vi "20T_Go_To_Set.vi"(8 "error in (no error)":errorcluster, 10 "20T Control":T1={"Clamp"=TRUE, "Switch Heater"=TRUE, "Go to Zero"=TRUE, "Go to Set"=FALSE, "Go to Hold"=FALSE, "Field Setpoint (T)"=3.4572, "Rate Setpoint (T/min)"=0.0, "Set Rate"=FALSE, "Activate lambda control"=FALSE, "Set lambda NV"=FALSE, "lambda NV  SP"=3.4572} {"lambda NV  SP" format="%.1f"; "Rate Setpoint (T/min)" format="%6_5f"; "Field Setpoint (T)" format="%#4_5f"}, 11 "Mercury Reference In":T2) -> (0 "error out":errorcluster)   [LabVIEW 2019]
uses:
  Equipment/Mercury iXX/Public/Controls/Mercury Reference.ctl
  Equipment/Mercury iXX/Public/Controls/Comms Transport Layer.ctl
  Equipment/Mercury iXX/Private/Controls/Query Dynamic Reference.ctl
  Monitor Communication/Gustav/20T_Control.ctl
  Global/Global Variables/Data_Display_global.vi
  Equipment/Mercury iXX/Public/Libraries/Magnet/Open/Open Magnet Device.vi
  Monitor Communication/sub-vis/20T_Open_Queue.vi
  Monitor Communication/sub-vis/20T_Queue_Commands.vi
  Equipment/Mercury iXX/Mercury iXX.lvlib
  Equipment/Mercury iXX/Public/Libraries/Magnet.lvlib
panel:
  # "20 T"
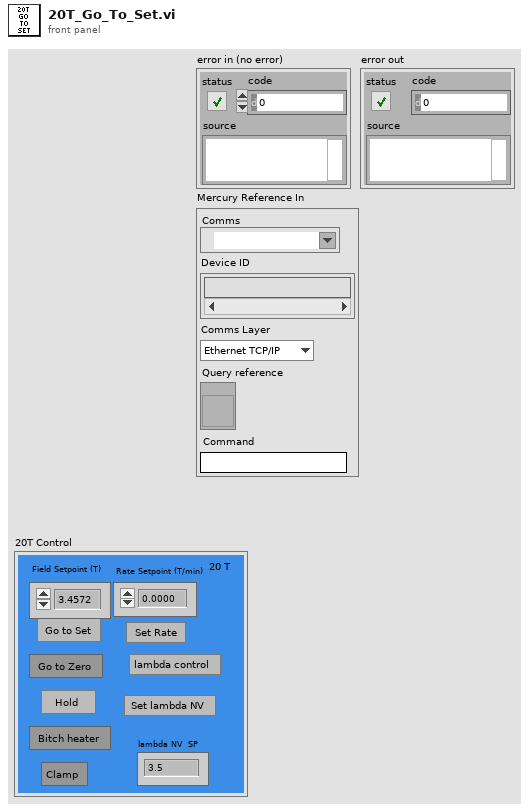
[diagram p1: front panel]
types:
  T1 = typedef "20T_Control.ctl" = cluster{"Clamp":bool, "Switch Heater":bool, "Go to Zero":bool, "Go to Set":bool, "Go to Hold":bool, "Field Setpoint (T)":dbl, "Rate Setpoint (T/min)":dbl, "Set Rate":bool, "Activate lambda control":bool, "Set lambda NV":bool, "lambda NV  SP":dbl}
  T2 = typedef "Mercury iXX.lvlib/Mercury Reference.ctl" = cluster{"Comms":refnum<visa-resource-name>, "Device ID":string[], "Comms Layer":T3, "Command":string, "Query reference":T4}
  T3 = typedef "Mercury iXX.lvlib/Comms Transport Layer.ctl" = enum16{"Ethernet TCP/IP", "USB", "ISOBus - RS-232", "GPIB"}
  T4 = typedef "Mercury iXX.lvlib/Query Dynamic Reference.ctl" = refnum<vi>
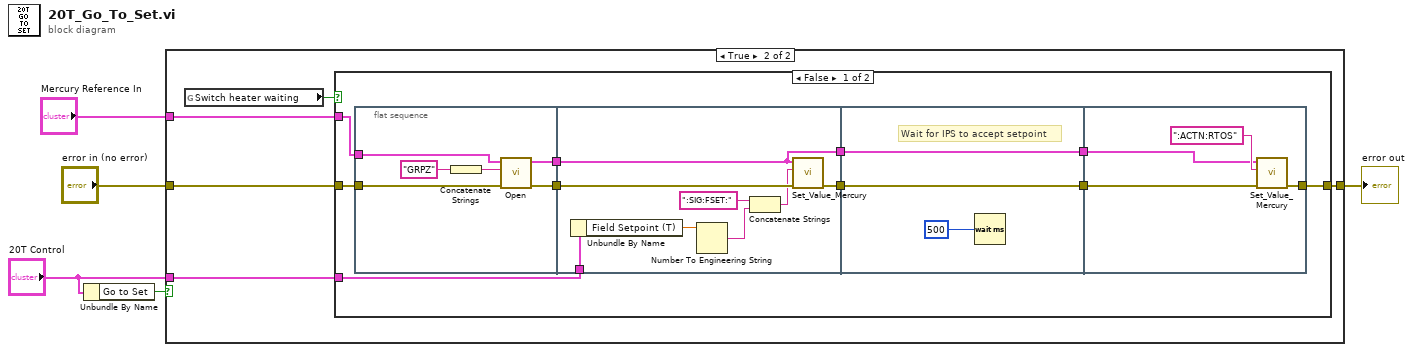
[diagram p0: block diagram]
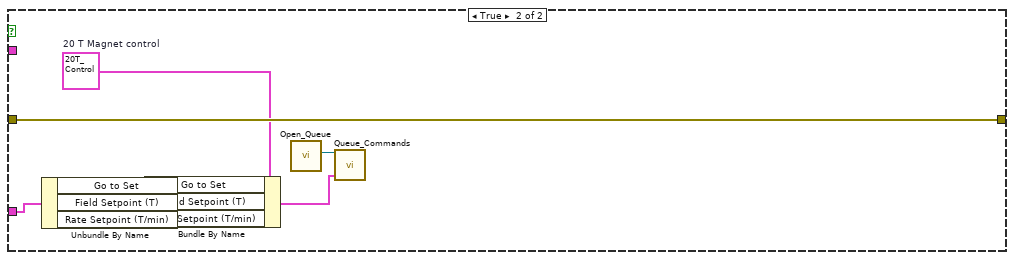
[diagram p3: hidden frame]
diagram:
  n1 = Unbundle By Name("20T Control") -> ("Go to Set"=w4:bool)
  n2 = case shown="True" w4 {
    tunnel: [w6 w7] -> w5
    tunnel: "20T Control" -> [_ w10]
    tunnel: "Mercury Reference In" -> [_ w9]
    tunnel: "error in (no error)" -> [w6 w8]
    frame False {
    }
    frame True {
      n3 = global read "Data_Display_global.vi" "Switch heater waiting"() -> (w11:bool)
      n4 = case shown="False" w11 {
        tunnel: [w21 w49] -> w7
        tunnel: w10 -> [w20 w48]
        tunnel: w9 -> [w17 _]
        tunnel: w8 -> [w16 w49]
        frame False {
          n5 = flat-sequence {
            tunnel: [w22] -> w19
            tunnel: [w23] -> w18
            tunnel: w17 -> [w25]
            tunnel: w16 -> [w24]
            tunnel: [w31] -> w15
            tunnel: [w33] -> w13
            tunnel: w20 -> [w28]
            tunnel: w19 -> [w32]
            tunnel: w18 -> [w33]
            tunnel: w15 -> [w38]
            tunnel: [w38] -> w14
            tunnel: w13 -> [w37]
            tunnel: [w37] -> w12
            tunnel: [w41] -> w21
            tunnel: w14 -> [w39]
            tunnel: w12 -> [w40]
            frame #0 {
              n6 = Concatenate Strings("GRPZ" ("Device Identifier")) -> (w27:string)
              n7 = call-poly "Open.vi"("error in (no error)"=w24, "Device Identifier"=w27, "Mercury Reference In"=w25) -> ("error out"=w22:errorcluster, "Mercury Reference Out"=w23:T2)  [unwired: 1 in, 6 out]
            }
            frame #1 {
              n8 = Unbundle By Name(w28) -> ("Field Setpoint (T)"=w29:dbl)
              n9 = Number To Engineering String(4:w29) -> (0:w35:string)  [unwired: 3 in]
              n10 = Concatenate Strings(":SIG:FSET:", w35) -> (w30:string)
              n11 = call "Set_Value_Mercury.vi"("error in"=w32, "Noun(s)"=w30, "Mercury Reference In"=w33) -> ("error out"=w31:errorcluster)  [unwired: 7 in, 1 out]
            }
            frame #2 {
              # "Wait for IPS to accept setpoint"
              n12 = Wait (ms)(milliseconds to wait=500) -> ()  [unwired: 1 out]
            }
            frame #3 {
              n13 = call "Set_Value_Mercury.vi"("error in"=w39, "Noun(s)"=":ACTN:RTOS", "Mercury Reference In"=w40) -> ("error out"=w41:errorcluster)  [unwired: 7 in, 1 out]
            }
          }
        }
        frame True {
          w47 = T1 {"Clamp"=FALSE, "Switch Heater"=FALSE, "Go to Zero"=FALSE, "Go to Set"=FALSE, "Go to Hold"=FALSE, "Field Setpoint (T)"=3.4572, "Rate Setpoint (T/min)"=0.0, "Set Rate"=FALSE, "Activate lambda control"=FALSE, "Set lambda NV"=FALSE, "lambda NV  SP"=3.4572}  # 20 T Magnet control
          n14 = Unbundle By Name(w48) -> ("Go to Set"=w45:bool, "Field Setpoint (T)"=w44:dbl, "Rate Setpoint (T/min)"=w43:dbl)
          n15 = Bundle By Name(cluster=w47, "Go to Set"=w45, "Field Setpoint (T)"=w44, "Rate Setpoint (T/min)"=w43) -> (w46:T1)
          n16 = call-poly "Open_Queue.vi"() -> ("queue out"=w50:refnum<queue>)  [unwired: 10 in, 1 out]
          n17 = call-poly "Queue_Commands.vi"("20T Control (in)"=w46, "20T Queue"=w50) -> ()  [unwired: 1 in, 1 out]
        }
      }
    }
  }
  "error out" <- w5
